vi "SubPanel.vi"(8 "error in (no error)":errorcluster, 10 "Data":variant, 11 "Detector Manager in":refnum<class "Detector Manager.lvclass">) -> (0 "error out":errorcluster, 3 "Detector Manager out":refnum<class "Detector Manager.lvclass">)   [LabVIEW 2026, in "TALOS.lvlib" / "Detector Manager.lvlib" / "Detector Manager.lvclass"]
doc: "Put in this VI the code to decode and display the data as generated in the corresponding HW class."
uses:
  Detector Manager.lvclass
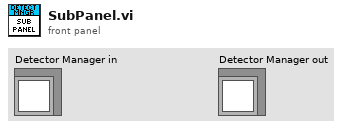
[diagram p1: front panel]
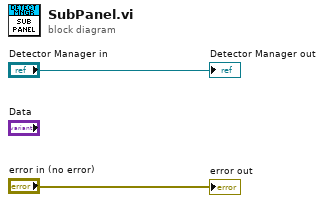
[diagram p0: block diagram]
diagram:
  "error out" <- "error in (no error)"
  "Detector Manager out" <- "Detector Manager in"
